vi "InitNet.vi"(10 "Hidden Neurons":dbl[](array[numeric]), 11 "Inputs":dbl) -> (3 "Neuron Stucture":T1)   [LabVIEW 2012]
uses:
  NeuronData.ctl
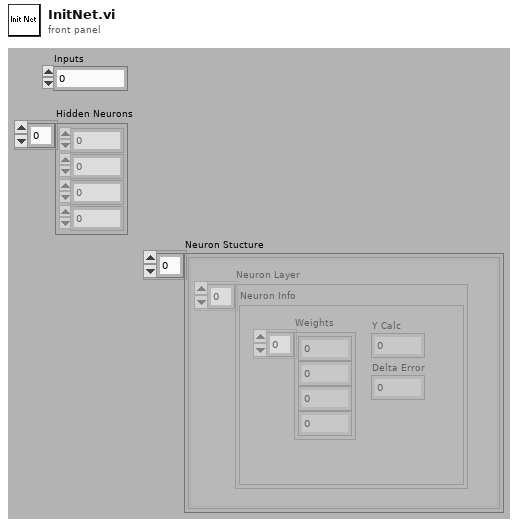
[diagram p1: front panel]
types:
  T1 = typedef "NeuronData.ctl" = cluster{"Neuron Layer":cluster{"Weights":dbl[], "Y Calc":dbl, "Delta Error":dbl}[]}[]
  T2 = cluster{cluster{dbl[], "Output":dbl, "Error":dbl}[]}
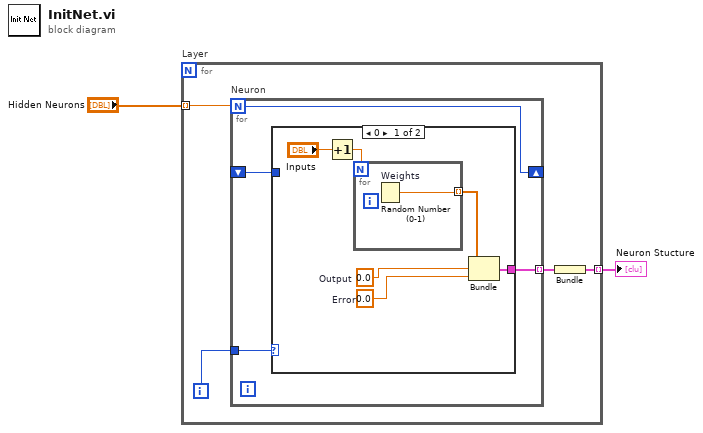
[diagram p0: block diagram]
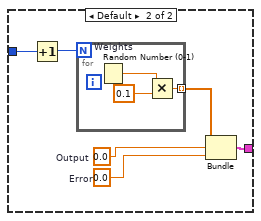
[diagram p2: hidden frame]
diagram:
  n1 = for "Layer" {
    tunnel: [w5] -> w1 mode=indexing
    tunnel: "Hidden Neurons" -> [w3] mode=indexing
    i -> [w4]
    n2 = for "Neuron" {
      N: w3 -> [w8]
      tunnel: [w10] -> w6 mode=indexing
      tunnel: w4 -> [w9]
      shift-right: [w8] -> _
      shift-left: _ -> [w7]
      n3 = case shown="0" w9 {
        tunnel: [w11 w18] -> w10
        tunnel: w7 -> [_ w21]
        frame 0 {
          w15 = 0.0  # Error
          w16 = 0.0  # Output
          n4 = Increment(x="Inputs") -> (x+1=w12:dbl)
          n5 = for {
            N: w12 -> [_]
            tunnel: [w17] -> w14 mode=indexing
            n6 = Random Number (0-1) "Weights"() -> (number: 0 to 1=w17:dbl)
          }
          n7 = Bundle(w14, "Output"=w16, "Error"=w15) -> (w11:cluster{dbl[], "Output":dbl, "Error":dbl})  [unwired: 1 in]
        }
        frame Default {
          w22 = 0.0  # Error
          w23 = 0.0  # Output
          n8 = Increment(x=w21) -> (x+1=w20:i32)
          n9 = for {
            N: w20 -> [_]
            tunnel: [w24] -> w19 mode=indexing
            n10 = Random Number (0-1) "Weights"() -> (number: 0 to 1=w26:dbl)
            n11 = Multiply(x=w26, y=0.1) -> (x*y=w24:dbl)
          }
          n12 = Bundle(w19, "Output"=w23, "Error"=w22) -> (w18:cluster{dbl[], "Output":dbl, "Error":dbl})  [unwired: 1 in]
        }
      }
    }
    n13 = Bundle(w6) -> (w5:T2)  [unwired: 1 in]
  }
  "Neuron Stucture" <- w1
